vi "Extract Analog Data.vi"(8 "error in (no error)":errorcluster, 10 "Analog Data In":sgl[][](array[numeric]), 11 "FPGA Reference In":refnum<k20>) -> (0 "error out":errorcluster, 2 "Analog Data Out":sgl[][](array[numeric]), 3 "Analog Data":T1)   [LabVIEW 2020]
uses:
  Type Definitions/Analog Data.ctl
  <vilib>/Utility/error.llb/Error Cluster From Error Code.vi
  <vilib>/rvi/errors/niLvFpgaAdjustHostInterfaceError.vi
  <vilib>/rvi/interface/nirviReadWriteControl/nirviReadWriteControl.xnode
  NiFpgaLv.dll
  <vilib>/rvi/interface/Simulation/niFpgaSimulationCallBeginRW.vi
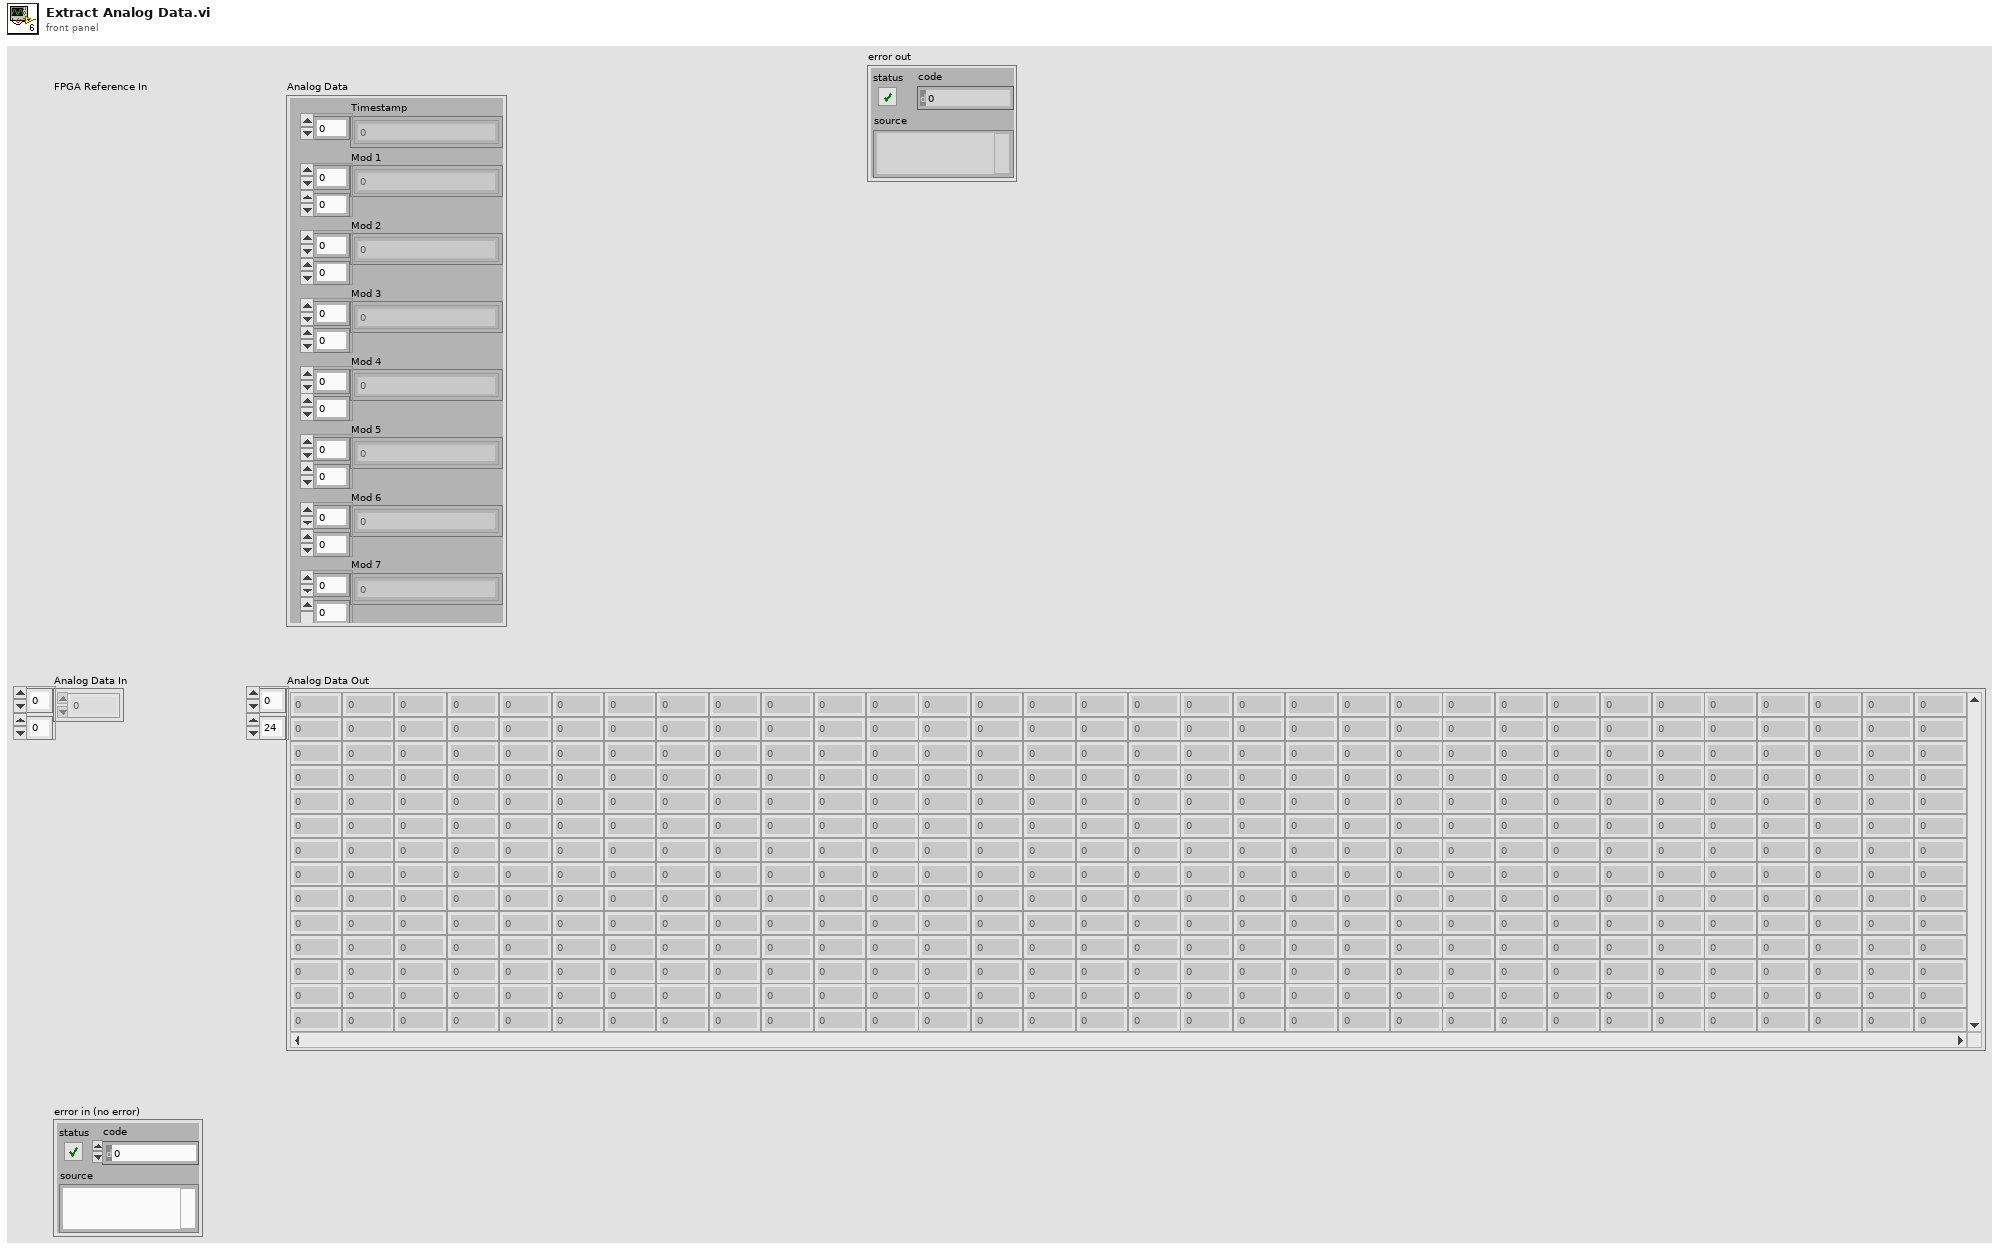
[diagram p1: front panel]
types:
  T1 = typedef "Analog Data.ctl" = cluster{"Timestamp":dbl[], "Mod 1":sgl[][], "Mod 2":sgl[][], "Mod 3":sgl[][], "Mod 4":sgl[][], "Mod 5":sgl[][], "Mod 6":sgl[][], "Mod 7":sgl[][]}
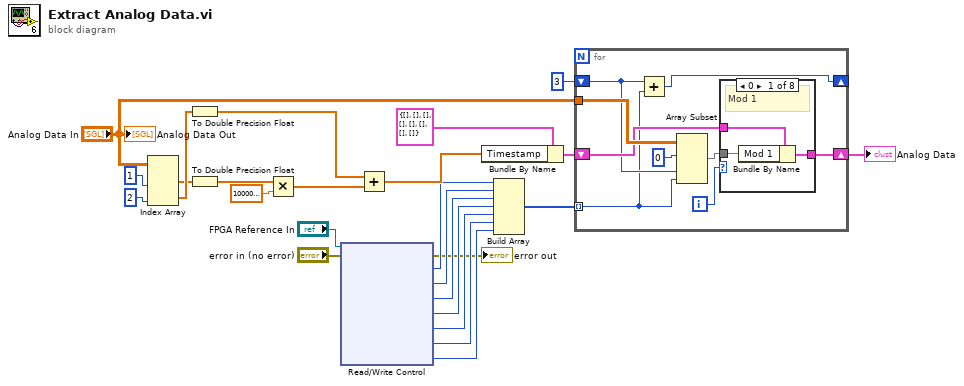
[diagram p0: block diagram]
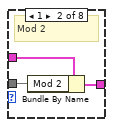
[diagram p2: hidden frame]
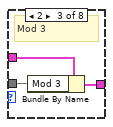
[diagram p3: hidden frame]
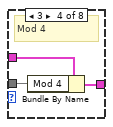
[diagram p4: hidden frame]
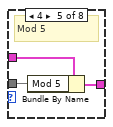
[diagram p5: hidden frame]
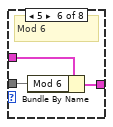
[diagram p6: hidden frame]
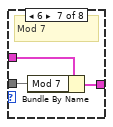
[diagram p7: hidden frame]
diagram:
  n1 = Index Array(array="Analog Data In", index (col) #1=1 ("disabled index (col)"), index (col) #2=2 ("index (row)")) -> (element #1=w17:sgl[], element #2=w19:sgl[])  [unwired: 2 in]
  n2 = To Double Precision Float(number=w19) -> (double precision float=w20:dbl[])
  n3 = To Double Precision Float(number=w17) -> (double precision float=w18:dbl[])
  n4 = Multiply(x=w18, y=1000000000.0) -> (x*y=w16:dbl[])
  n5 = xnode "Read/Write Control"("FPGA VI Reference In"="FPGA Reference In", "error in"="error in (no error)") -> ("error out"=→"error out":errorcluster, "Mod 1 Length"=w2:i32, "Mod 2 Length"=w3:i32, "Mod 3 Length"=w4:i32, "Mod 4 Length"=w5:i32, "Mod 5 Length"=w6:i32, "Mod 6 Length"=w7:i32, "Mod 7 Length"=w8:i32)  [unwired: 1 out]
  n6 = Add(x=w20, y=w16) -> (x+y=w21:dbl[])
  n7 = Bundle By Name(cluster=T1 {"Timestamp"=[], "Mod 1"=[], "Mod 2"=[], "Mod 3"=[], "Mod 4"=[], "Mod 5"=[], "Mod 6"=[], "Mod 7"=[]} ("Analog Data"), "Timestamp"=w21) -> (w12:T1)
  n8 = Build Array(w2, w3, w4, w5, w6, w7, w8) -> (w9:i32[])
  n9 = for {
    tunnel: w9 -> [w27] mode=indexing
    tunnel: "Analog Data In" -> [w34]
    shift-right: [w33] -> _
    shift-left: 3 ("index") -> [w28]
    shift-right: [w29] -> w22
    shift-left: w12 -> [w31]
    i -> [w32]
    n10 = Add(x=w28, y=w27) -> (x+y=w33:i32)
    n11 = Array Subset(array=w34, index (row)=0 ("index"), index (col)=w28, length (col)=w27) -> (w30:sgl[][])  [unwired: 1 in]
    n12 = case shown="0" w32 {
      tunnel: w31 -> [w37 w40 w43 w46 w49 w52 w55 w56]
      tunnel: w30 -> [w36 w39 w42 w45 w48 w51 w54 _]
      tunnel: [w35 w38 w41 w44 w47 w50 w53 w56] -> w29
      frame 0 {
        # "Mod 1"
        n13 = Bundle By Name(cluster=w37, "Mod 1"=w36) -> (w35:T1)
      }
      frame 1 {
        # "Mod 2"
        n14 = Bundle By Name(cluster=w40, "Mod 2"=w39) -> (w38:T1)
      }
      frame 2 {
        # "Mod 3"
        n15 = Bundle By Name(cluster=w43, "Mod 3"=w42) -> (w41:T1)
      }
      frame 3 {
        # "Mod 4"
        n16 = Bundle By Name(cluster=w46, "Mod 4"=w45) -> (w44:T1)
      }
      frame 4 {
        # "Mod 5"
        n17 = Bundle By Name(cluster=w49, "Mod 5"=w48) -> (w47:T1)
      }
      frame 5 {
        # "Mod 6"
        n18 = Bundle By Name(cluster=w52, "Mod 6"=w51) -> (w50:T1)
      }
      frame 6 {
        # "Mod 7"
        n19 = Bundle By Name(cluster=w55, "Mod 7"=w54) -> (w53:T1)
      }
      frame Default {
        # "Mod 7"
      }
    }
  }
  "Analog Data" <- w22
  "Analog Data Out" <- "Analog Data In"
